vi "11.Evd.4_Ask2.vi"() -> ()   [LabVIEW 2025]
panel:
  in  "Stop Button":bool
  in  "Initial temperature in C":dbl
  out "Kelvin":dbl
  out "Celsius":dbl
  out "Fahrenheit":dbl
  out "Kelvin":dbl(slide) scale=0.0..500.0
  out "Celsius":dbl(slide) scale=-200.0..200.0
  out "Fahrenheit":dbl(slide) scale=-300.0..300.0
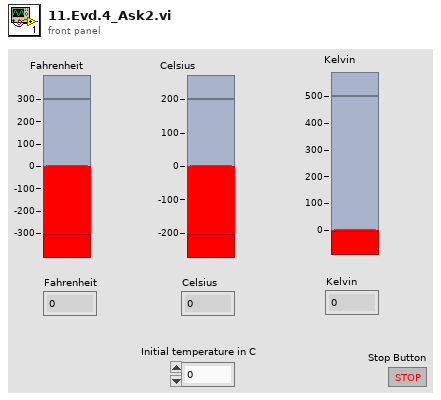
[diagram p1: front panel]
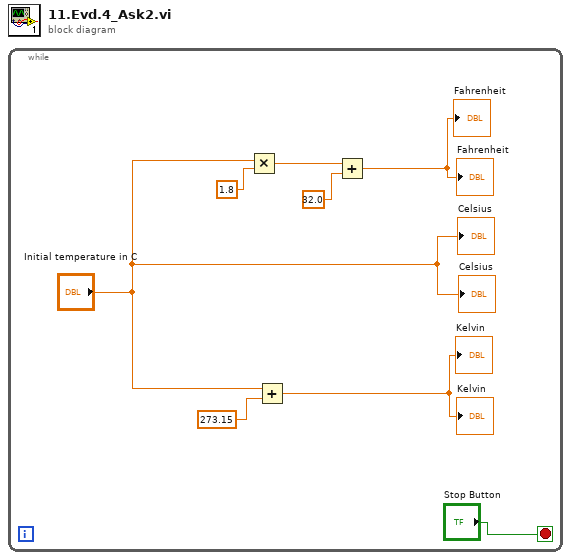
[diagram p0: block diagram]
diagram:
  n1 = while {
    stop <- "Stop Button" stop-if-true
    n2 = Multiply(x="Initial temperature in C", y=1.8) -> (x*y=w6:dbl)
    n3 = Add(x="Initial temperature in C", y=273.15) -> (x+y=→"Kelvin" →"Kelvin":dbl)
    n4 = Add(x=w6, y=32.0) -> (x+y=→"Fahrenheit" →"Fahrenheit":dbl)
    "Celsius" <- "Initial temperature in C"
    "Celsius" <- "Initial temperature in C"
  }
